vi "check diagnostics.vi"(8 "error in":errorcluster, 10 "data dictionary in":refnum<class "data dictionary.lvclass">, 11 "Profibus Module configuration in":refnum<class "Profibus Module configuration.lvclass">) -> (0 "error out":errorcluster, 3 "diagnostics":T1[](array[typedef]))   [LabVIEW 2013, in "Profibus Module runtime.lvclass"]
uses:
  Profibus Module runtime.lvclass
  <vilib>/NI/Tag Bus/dictionary/data dictionary.lvclass
  configuration/Profibus Module configuration.lvclass
  profibus diagnostics reporting.ctl
  configuration/error throw specification.ctl
  configuration/Profibus Module configuration.lvclass/Profibus Module configuration.ctl
  <vilib>/NI/Tag Bus/tag/tag descriptor.lvclass/tag descriptor.ctl
  <vilib>/NI/Tag Bus/dictionary/data dictionary.lvclass/data dictionary.ctl
  <vilib>/NI/Tag Bus/dictionary/lookup polymorphs/locate Array of U8.vi
  <vilib>/NI/Tag Bus/dictionary/search/find data index.vi
  <vilib>/NI/Tag Bus/dictionary/search/search string list.vi
  <vilib>/NI/Tag Bus/dictionary/tag not found.vi
  <vilib>/NI/Tag Bus/tag/tag descriptor.lvclass
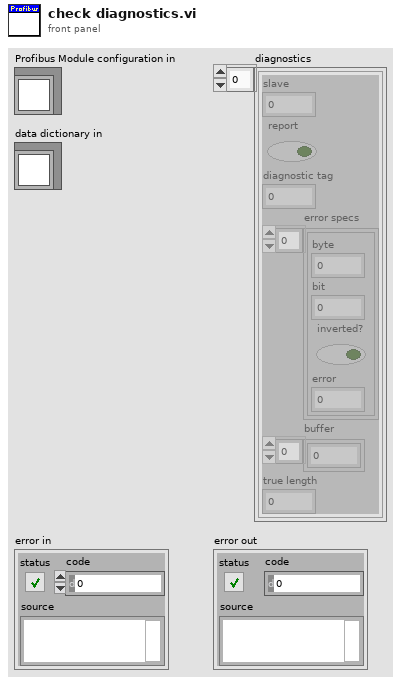
[diagram p1: front panel]
types:
  T1 = typedef "Profibus Module runtime.lvclass/profibus diagnostics reporting.ctl" = cluster{"slave":i8, "report":bool, "diagnostic tag":i32, "error specs":T2[], "buffer":u8[], "true length":u8}
  T2 = typedef "Profibus Module configuration.lvclass/error throw specification.ctl" = cluster{"byte":i32, "bit":i32, "inverted?":bool, "error":i32}
  T3 = typedef "Profibus Module configuration.lvclass/slave diagnostic configuration.ctl" = cluster{"slave":i8, "report":bool, "channel":refnum<class "TBM channel.lvclass">, "error specs":T2[]}
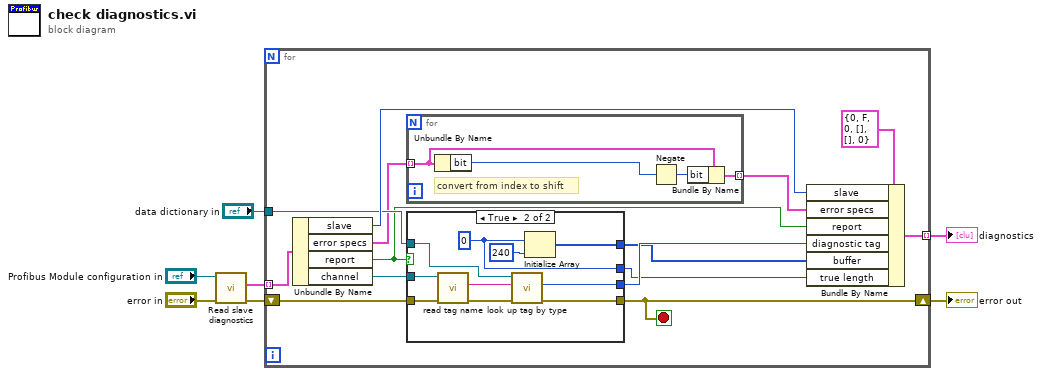
[diagram p0: block diagram]
diagram:
  n1 = call "Read slave diagnostics.vi"("error in"="error in", "Profibus Module configuration in"="Profibus Module configuration in") -> ("error out"=w4:errorcluster, "slave diagnostics"=w5:T3[])  [unwired: 7 in, 1 out]
  n2 = for {
    tunnel: w5 -> [w21] mode=indexing
    shift-right: [w13] -> w3
    shift-left: w4 -> [w17]
    tunnel: [w19] -> w2 mode=indexing
    tunnel: "data dictionary in" -> [w15]
    stop <- w13 stop-if-true
    n3 = Unbundle By Name(w21) -> ("slave"=w18:i8, "error specs"=w11:T2[], "report"=w12:bool, "channel"=w16:refnum<class "TBM channel.lvclass">)
    n4 = for {
      tunnel: w11 -> [w25] mode=indexing
      tunnel: [w24] -> w10 mode=indexing
      # "convert from index to shift"
      n5 = Unbundle By Name(w25) -> ("bit"=w23:i32)
      n6 = Negate(x=w23) -> (-x=w22:i32)
      n7 = Bundle By Name(cluster=w25, "bit"=w22) -> (w24:T2)
    }
    n8 = case shown="True" w12 {
      tunnel: w17 -> [w26 w33]
      tunnel: w16 -> [_ w32]
      tunnel: w15 -> [_ w36]
      tunnel: [w26 w35] -> w13
      tunnel: [_ w34] -> w14
      tunnel: [_ w28] -> w9
      tunnel: [_ w27] -> w8
      frame False {
      }
      frame True {
        w27 = u8 0
        n9 = call <vilib>:"read tag name.vi"("error in"=w33, "system tag in"=w32) -> ("error out"=w31:errorcluster, "name"=w30:string)  [unwired: 7 in, 1 out]
        n10 = call-poly <vilib>:"look up tag by type.vi"("error in"=w31, "name"=w30, "data dictionary in"=w36) -> ("error out"=w35:errorcluster, "index"=w34:i32)  [unwired: 6 in, 1 out]
        n11 = Initialize Array(w27, u8 240) -> (w28:u8[])
      }
    }
    n12 = Bundle By Name(cluster=T1 {"slave"=0, "report"=FALSE, "diagnostic tag"=0, "error specs"=[], "buffer"=[], "true length"=0} ("diagnostics settings"), "slave"=w18, "error specs"=w10, "report"=w12, "diagnostic tag"=w14, "buffer"=w9, "true length"=w8) -> (w19:T1)
  }
  "diagnostics" <- w2
  "error out" <- w3
